vi "concatenate strings.vi"() -> ()   [LabVIEW 2020]
panel:
  out "full name":string
  in  "last name":string
  in  "first name":string
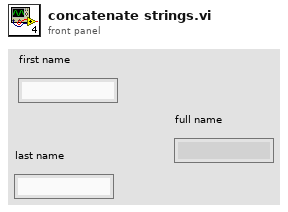
[diagram p1: front panel]
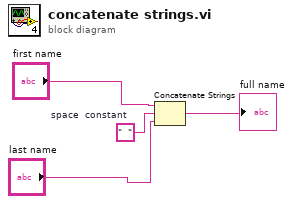
[diagram p0: block diagram]
diagram:
  w1 = "  "  # space  constant
  n1 = Concatenate Strings("first name", w1, "last name") -> (→"full name":string)
